vi "HK Channel Delete Item.vi"(8 "error in (no error)":errorcluster, 10 "Channel Name":string, 11 "HK Channel in":refnum<class "HK Table.lvclass">) -> (0 "error out":errorcluster, 1 "Deleted?":bool, 2 "Deleted Item":refnum<class "HK Item.lvclass">, 3 "HK Channel out":refnum<class "HK Table.lvclass">)   [LabVIEW 2019, in "HK Table.lvclass"]
uses:
  HK Table.lvclass
  HK Item/HK Item.lvclass
  HK Table.lvclass/HK Table.ctl
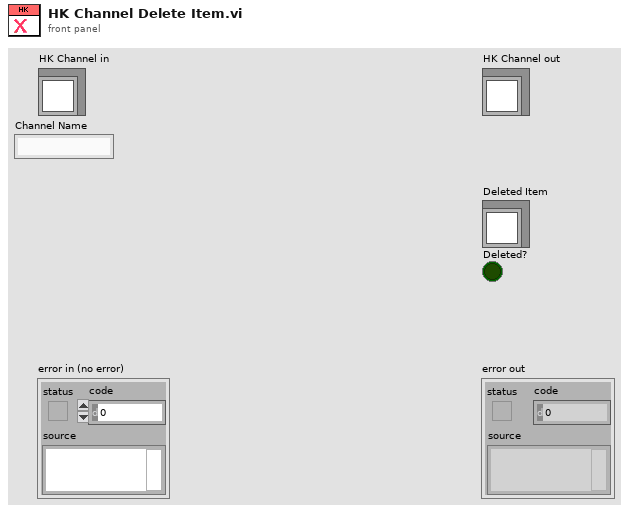
[diagram p1: front panel]
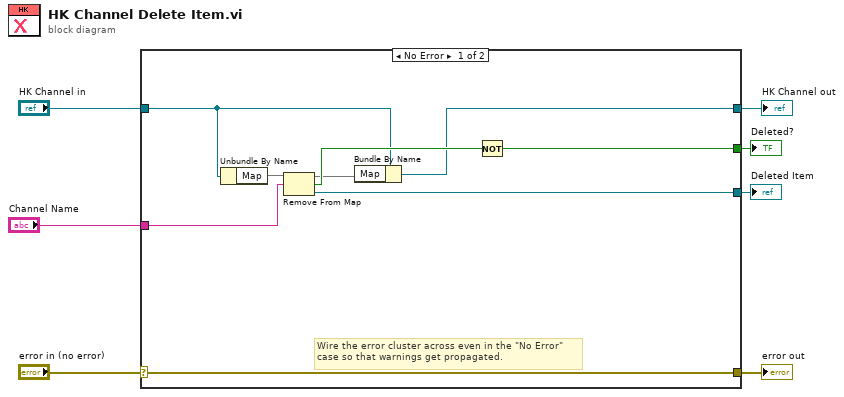
[diagram p0: block diagram]
diagram:
  n1 = case shown="No Error" "error in (no error)" {
    selector: "error in (no error)" -> [w16 w18]
    tunnel: [w16 w18] -> w6
    tunnel: [w9 w17] -> w4
    tunnel: "HK Channel in" -> [w8 w17]
    tunnel: "Channel Name" -> [w14 _]
    tunnel: [w13 _] -> w2
    tunnel: [w11 _] -> w1
    frame No Error {
      # "Wire the error cluster across even in the \"No Error\"\ncase so that warnings get propagated."
      n2 = Unbundle By Name(w8) -> ("Map"=w15:map{string, refnum<class "HK Item.lvclass">})
      n3 = Remove From Map(10:w14, 11:w15) -> (1:w13:refnum<class "HK Item.lvclass">, 2:w12:bool, 3:w10:map{string, refnum<class "HK Item.lvclass">})
      n4 = Bundle By Name(cluster=w8, "Map"=w10) -> (w9:refnum<class "HK Table.lvclass">)
      n5 = Not(x=w12) -> (.not. x?=w11:bool)
    }
    frame Error {
    }
  }
  "error out" <- w6
  "HK Channel out" <- w4
  "Deleted Item" <- w2
  "Deleted?" <- w1
